vi "get compatible resources as tree items.vi"(8 "error in (no error)":errorcluster, 10 "Tree Refnum":refnum<vi>, 11 "Item Ref in":T1 format="%.0x") -> (0 "error out":errorcluster, 3 "Item Ref out":T1 format="%.0x")   [LabVIEW 2016, in "FPGA RM System Definition API.lvlib"]
uses:
  FPGA-Resource-Manager-APIs/Source/System Definition/FPGA RM System Definition API.lvlib
  <vilib>/NI Veristand/Custom Device API/Custom Device Item Ref.ctl
  <vilib>/NI VeriStand/Custom Device API/Custom Device API.lvlib
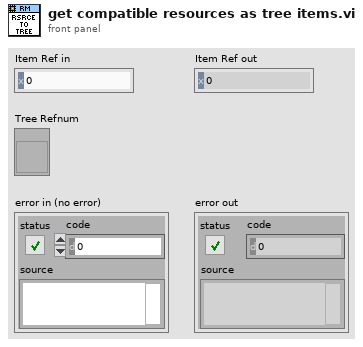
[diagram p1: front panel]
types:
  T1 = typedef "Custom Device API.lvlib/Custom Device Item Ref.ctl" = u64
  T2 = cluster{"Left Cell String":string, "Child Text":string[], "Child Tag":string, "Item Indent":i32, "Child Only?":bool, "Glyph Index":i32}
  T3 = typedef "FPGA RM System Definition API.lvlib/Channel Type.ctl" = enum16{"Write Channel", "Read Channel", "Write Waveform", "Read Waveform"}
  T4 = typedef "FPGA RM System Definition API.lvlib/fpga resource.ctl" = cluster{"name":string, "datatype":string, "channel type":T3, "value":variant, "notes":string}
  T5 = cluster{"Left Cell String":string, "Child Text":string[], "Child Tag":string, "Item Indent":i32, "Child Only?":bool, "Glyph Index":i32}[]
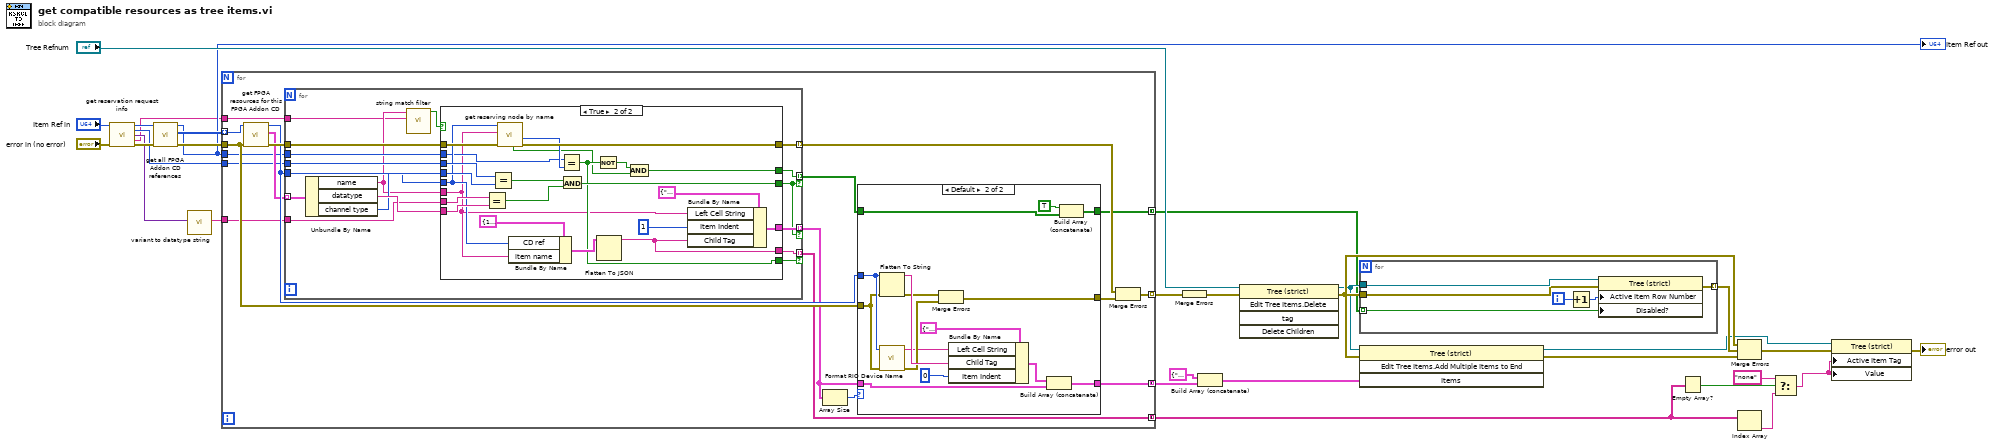
[diagram p0: block diagram]
diagram:
  n1 = call "get reservation request info.vi"("Item Ref in"="Item Ref in", "error in (no error)"="error in (no error)") -> ("Item Ref out"=w21:T1, "channel type"=w17:T3, "datatype"=w15:variant, "Pattern"=w9:string, "error out"=w18:errorcluster)  [unwired: 9 in]
  n2 = call "get all FPGA Addon CD references.vi"("error in (no error)"=w18, "Item Ref in"=w21) -> ("error out"=w29:errorcluster, "FPGA Addon CD refs out"=w30:T1[], "Item Ref out"=w13:T1)  [unwired: 7 in]
  "Item Ref out" <- w13
  n3 = call "variant to datatype string.vi"("Variant"=w15) -> ("datatype string"=w14:string)  [unwired: 9 in, 1 out]
  n4 = for {
    tunnel: w14 -> [w36]
    tunnel: w30 -> [w34] mode=indexing
    tunnel: [w48] -> w8 mode=concatenating
    tunnel: [w38] -> w20 mode=concatenating
    tunnel: w29 -> [w47]
    tunnel: [w44] -> w28 mode=indexing
    tunnel: w17 -> [w35]
    tunnel: w13 -> [w33]
    tunnel: [w32] -> w5 mode=concatenating
    tunnel: w9 -> [w31]
    n5 = call "get FPGA resources for this FPGA Addon CD.vi"("error in (no error)"=w47, "Item Ref in"=w34) -> ("error out"=w46:errorcluster, "fpga resources"=w41:T4[], "Item Ref out"=w43:T1)  [unwired: 6 in, 1 out]
    n6 = for {
      tunnel: w41 -> [w81] mode=indexing
      tunnel: [w78] -> w37 mode=indexing if=w77
      tunnel: w43 -> [w74]
      tunnel: [w70] -> w39 mode=indexing if=w77
      tunnel: w46 -> [w83]
      tunnel: [w82] -> w45 mode=indexing
      tunnel: w36 -> [w76]
      tunnel: w35 -> [w75]
      tunnel: w33 -> [w73]
      tunnel: [w72] -> w32 mode=indexing if=w71
      tunnel: w31 -> [w68]
      n7 = Unbundle By Name(w81) -> ("name"=w69:string, "datatype"=w80:string, "channel type"=w79:T3)
      n8 = call "string match filter.vi"("string filter value"=w68, "string value"=w69) -> ("match?"=w67:bool)  [unwired: 9 in]
      n9 = case shown="True" w67 {
        tunnel: w83 -> [w84 w103]
        tunnel: [w84 w102] -> w82
        tunnel: w80 -> [_ w101]
        tunnel: w79 -> [_ w100]
        tunnel: [_ w99] -> w78
        tunnel: [_ w98] -> w77
        tunnel: w76 -> [_ w97]
        tunnel: w75 -> [_ w96]
        tunnel: w74 -> [_ w94]
        tunnel: w73 -> [_ w91]
        tunnel: [_ w90] -> w72
        tunnel: [_ w89] -> w71
        tunnel: [_ w87] -> w70
        tunnel: w69 -> [_ w85]
        frame False {
        }
        frame True {
          n10 = Equal?(x=w97, y=w101) -> (x = y?=w106:bool)
          n11 = Equal?(x=w96, y=w100) -> (x = y?=w107:bool)
          n12 = call "get reserving node by name.vi"("error in (no error)"=w103, "name"=w85, "Item Ref in"=w94) -> ("error out"=w102:errorcluster, "Dependent Node Ref"=w92:T1, "Found"=w88:bool)  [unwired: 5 in, 1 out]
          n13 = Bundle By Name(cluster=cluster{"CD ref":T1, "item name":string} {"CD ref"=18446744073709551615, "item name"=""}, "CD ref"=w94, "item name"=w85) -> (w93:cluster{"CD ref":T1, "item name":string})
          n14 = Equal?(x=w91, y=w92) -> (x = y?=w89:bool)
          n15 = And(x=w107, y=w106) -> (x .and. y?=w98:bool)
          n16 = Not(x=w89) -> (.not. x?=w86:bool)
          n17 = Flatten To JSON(anything=w93) -> (JSON string=w90:string)  [unwired: 2 in, 1 out]
          n18 = And(x=w86, y=w88) -> (x .and. y?=w87:bool)
          n19 = Bundle By Name(cluster=T2 {"Left Cell String"="", "Child Text"=[], "Child Tag"="", "Item Indent"=0, "Child Only?"=FALSE, "Glyph Index"=0} ("Items"), "Left Cell String"=w85, "Item Indent"=1, "Child Tag"=w90) -> (w99:T2)
        }
      }
    }
    n20 = Array Size(array=w37) -> (size(s)=w40:i32)
    n21 = case shown="Default" w40 {
      tunnel: [w51 w63] -> w48
      tunnel: w47 -> [w50 w57]
      tunnel: w43 -> [_ w61]
      tunnel: [w50 w58] -> w42
      tunnel: w37 -> [w51 w53]
      tunnel: w39 -> [w49 w56]
      tunnel: [w49 w55] -> w38
      frame 0 {
      }
      frame Default {
        n22 = Flatten To String(anything=w61, error in (no error)=w57) -> (data string=w65:string, error out=w60:errorcluster)  [unwired: 2 in, 1 out]
        n23 = call "Format RIO Device Name.vi"("error in (no error)"=w57, "FPGA CD Ref"=w61) -> ("error out"=w59:errorcluster, "String"=w52:string)  [unwired: 8 in]
        n24 = Merge Errors(w60, w59) -> (w58:errorcluster)
        n25 = Bundle By Name(cluster=T2 {"Left Cell String"="", "Child Text"=[], "Child Tag"="", "Item Indent"=0, "Child Only?"=FALSE, "Glyph Index"=0} ("Items"), "Left Cell String"=w52, "Child Tag"=w65, "Item Indent"=0) -> (w62:T2)
        n26 = Build Array (concatenate)(w62, w53) -> (w63:T5)
        n27 = Build Array (concatenate)(TRUE, w56) -> (w55:bool[])
      }
    }
    n28 = Merge Errors(w45, w42) -> (w44:errorcluster)
  }
  n29 = Merge Errors(w28) -> (w27:errorcluster)
  n30 = Build Array (concatenate)(T2 {"Left Cell String"="none", "Child Text"=[], "Child Tag"="", "Item Indent"=0, "Child Only?"=FALSE, "Glyph Index"=0} ("element"), w8) -> (w7:T5)
  n31 = invoke class="Tree (strict)" method="Edit Tree Items.Delete"(reference="Tree Refnum", error in=w27) -> (reference out=w22:refnum<vi>, error out=w24:errorcluster)  [unwired: 3 in, 3 out]
  n32 = for {
    tunnel: w20 -> [w112] mode=indexing
    tunnel: w22 -> [w111]
    tunnel: w24 -> [w110]
    tunnel: [w109] -> w26 mode=indexing
    i -> [w113]
    n33 = Increment(x=w113) -> (x+1=w108:i32)
    n34 = property on="Property Node" class="Tree (strict)"(reference=w111, error in=w110, "Active Item Row Number"=w108, "Disabled?"=w112) -> (error out=w109:errorcluster)  [unwired: 1 out]
  }
  n35 = invoke on="Invoke Node" class="Tree (strict)" method="Edit Tree Items.Add Multiple Items to End"(reference=w22, error in=w24, "Items"=w7) -> (reference out=w11:refnum<vi>, error out=w25:errorcluster)  [unwired: 1 in, 2 out]
  n36 = Empty Array?(array=w5) -> (empty?=w4:bool)
  n37 = Merge Errors(w24, w26, w25) -> (w12:errorcluster)
  n38 = Index Array(array=w5) -> (element=w3:string)  [unwired: 1 in]
  n39 = Select(t="none", s=w4, f=w3) -> (s? t:f=w2:string)
  n40 = property on="Property Node" class="Tree (strict)"(reference=w11, error in=w12, "Active Item Tag"=w2, "Value"=w2) -> (error out=→"error out":errorcluster)  [unwired: 1 out]
